vi "Habid_2-D_Histogram_Beta.vi"() -> ()   [LabVIEW 2009]
uses:
  <vilib>/Utility/file.llb/Write To Spreadsheet File (DBL).vi
  <vilib>/Analysis/3filter.llb/Butterworth Filter (DBL).vi
  <vilib>/Analysis/NI_AALBase.lvlib
  <vilib>/Analysis/NI_AALPro.lvlib
panel:
  in  "Save 2-D":bool
  in  "Result File Dir 2":path
  in  "Result File Name 2":string="1D_Histogram.txt"
  in  "Piezo Factor":dbl=0.88881
  out "SD":dbl[](array[numeric])
  in  "High Voltage Gain":dbl=5.0
  out "y-axis":dbl[](array[numeric])
  out "x-axis":dbl[](array[numeric])
  in  "Ramp Rate":dbl=5.0
  out "fit for M.A.":cluster{"Value":dbl, dbl, dbl[]}(graph)
  in  "Average Max?":bool
  out "Individual 2D Histogram":dbl[][](graph)
  out "Total 2D Histogram":dbl[][](graph)
  out "threshold":cluster{dbl, dbl, ext[]}(graph)
  out "Gain Multiplier I(t)":cluster{dbl, dbl, "Filtered X":dbl[]}(graph)
  out "After I(t)":cluster{dbl, dbl, "Filtered X":dbl[]}(graph)
  out "Before I(t)":cluster{dbl, "SamplingTime":dbl, "Data":ext[]}(graph)
  in  "start path":path=path "J:/data"
  out "NormAC":dbl[](array[numeric])
  in  "Save Curve?":bool
  out "CurrentFileName":string
  in  "Result File Name":string="1D_Histogram.txt"
  in  "Result File Dir":path
  in  "Save 1-D":bool
  out "SelectedCurves":i32
  out "CurvesInHistogram":bool[](array[boolean])
  in  "1-D Histogram?":bool
  in  "Continuous?":bool
  in  "Add Histogram?":bool
  in  "Beta bins":i32=100
  in  "Beta max":dbl=20.0
  in  "Beta min":dbl
  in  "Distance bins":i32=500
  in  "Distance max":dbl=4.0
  in  "Distance min":dbl
  in  "+/-":bool=TRUE
  out "DcData":dbl[](array[numeric])
  out "Beta":dbl[](array[numeric])
  out "DcDataLog":dbl[](array[numeric])
  out "TotalCurves":i32
  out "CurrentCurve":i32
  in  "Next Curve":bool
  in  "Previous Curve":bool
  out "AC I(t)":T1(graph)
  in  "Piezo Sensitivity (nm/V)":dbl=3.89
  in  "Z-mod Amp (V)":dbl=0.0257
  in  "Gac/Gdc":dbl=1.16618
  in  "low cutoff freq: fl":u32=600
  in  "high cutoff freq: fh":u32=1400
  out "DC I(t)":T2(graph)
  in  "DC cutoff freq":i32=1200
  out "Original I(t)":cluster{dbl, "SamplingTime":dbl, "Data":ext[]}(graph)
  out "DataBuffer":dbl[](array[numeric])
  out "Sampling Freq":dbl
  out "Sampling Time":dbl
  out "TimeLine":dbl[](array[numeric])
  in  "stop":bool
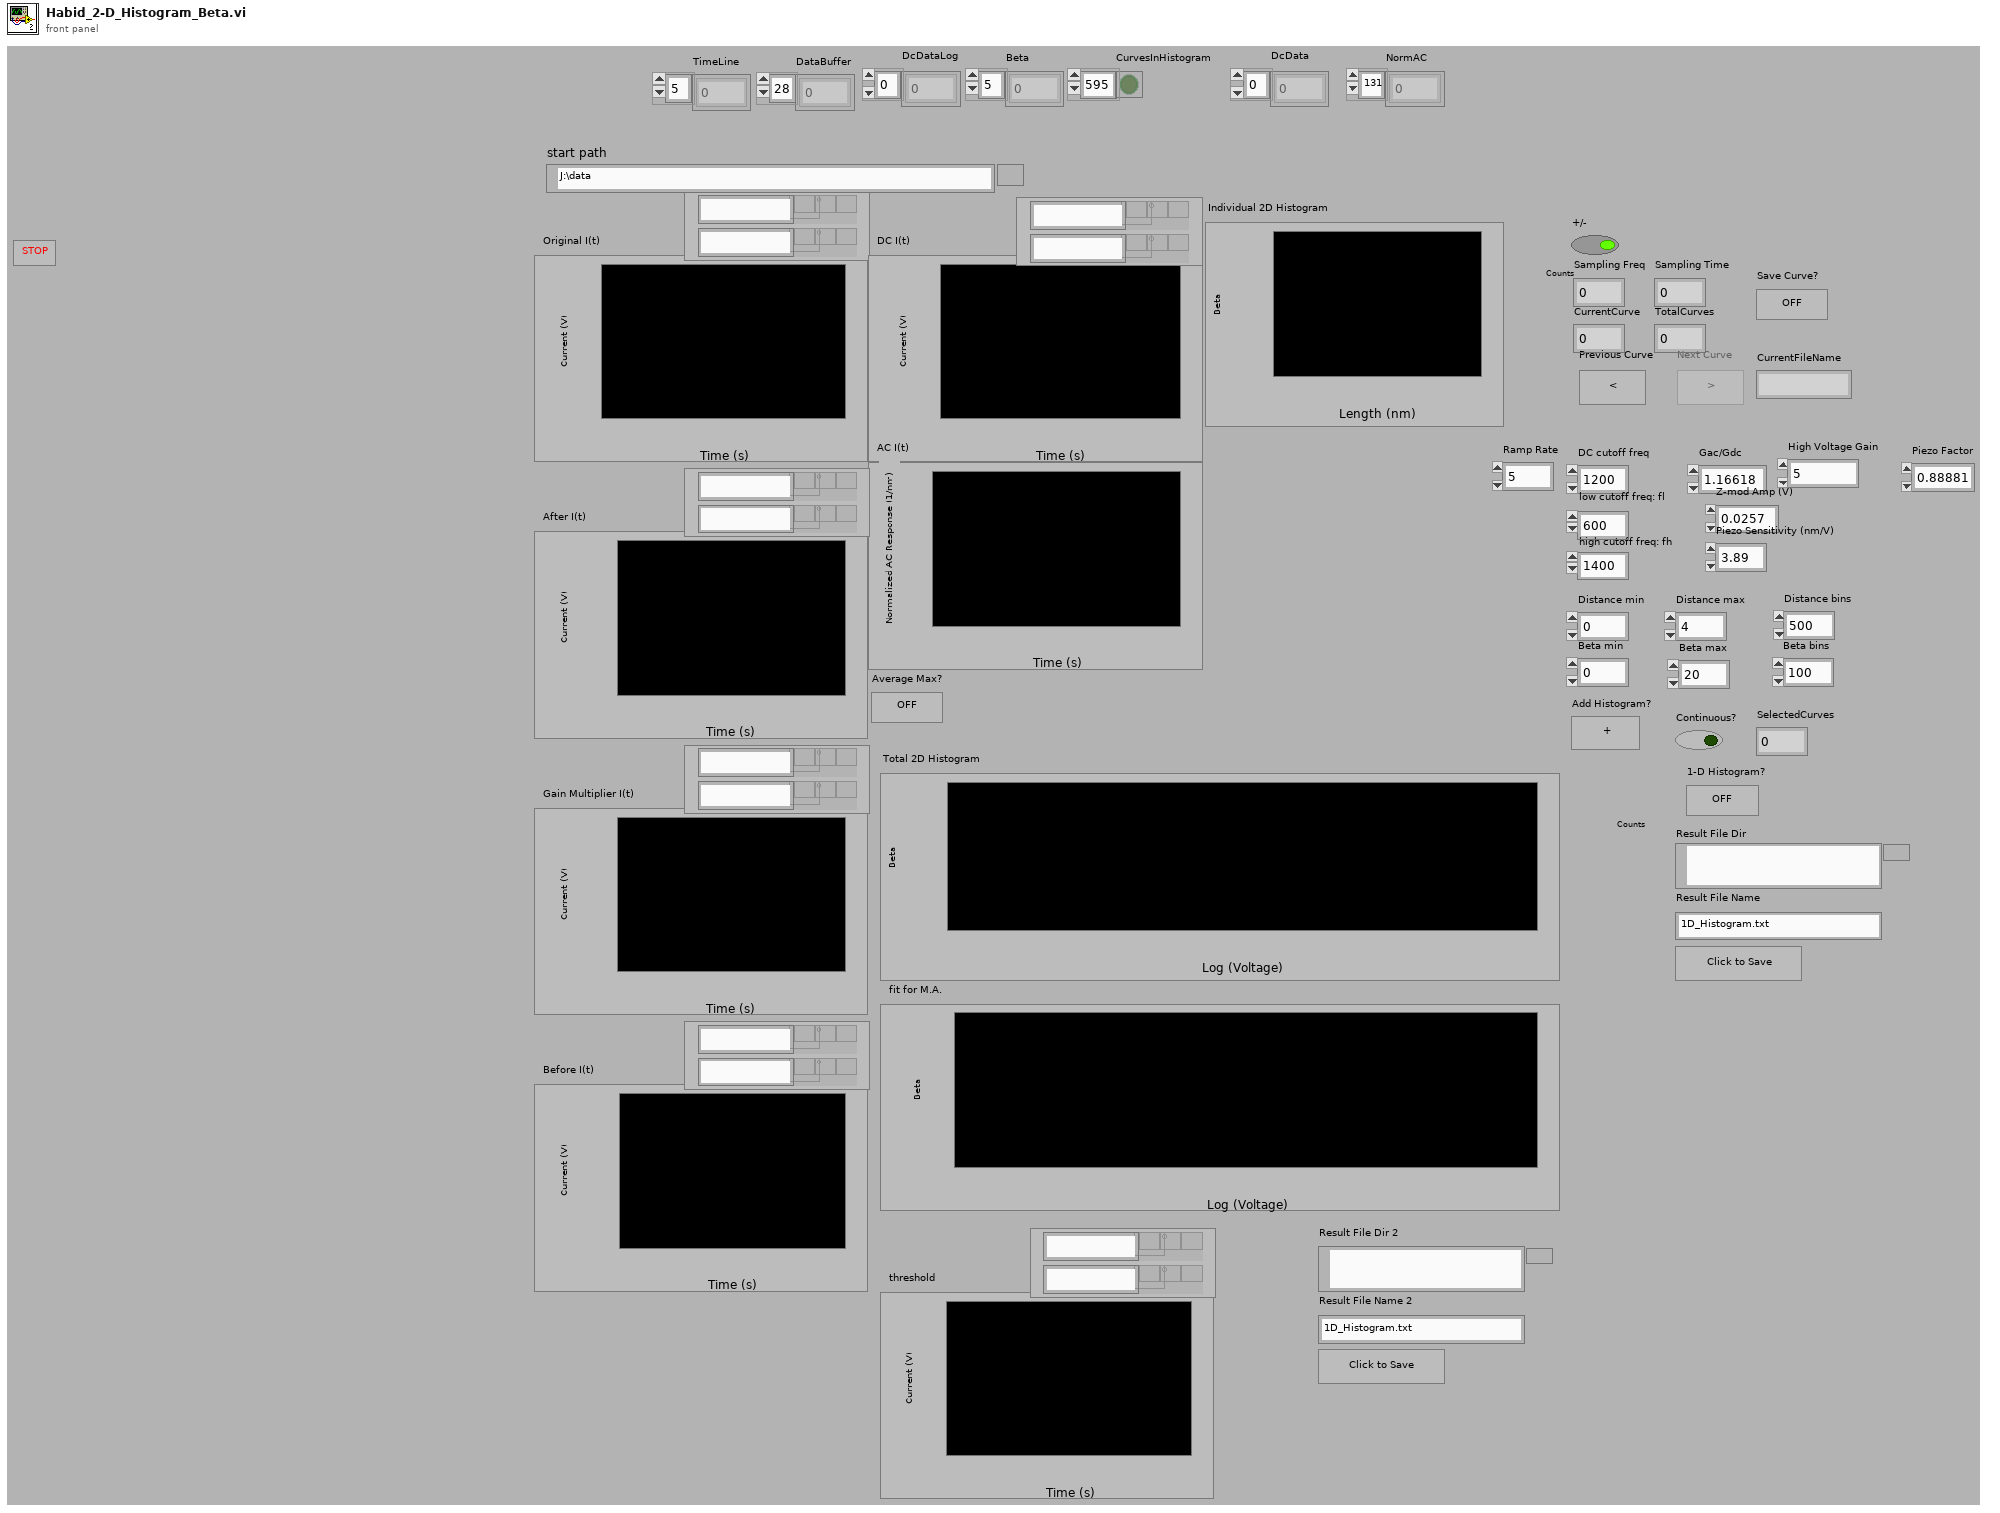
[diagram p1: front panel]
types:
  T1 = cluster{"Start Time":dbl, "Sampling Time":dbl, dbl[][]}
  T2 = cluster{dbl, "SamplingTime":dbl, "Filtered X":dbl[]}
  T3 = enum32{"Lowpass", "Highpass", "Bandpass", "Bandstop"}
  T4 = cluster{"Value":dbl, "XScale.Multiplier":dbl, dbl[]}
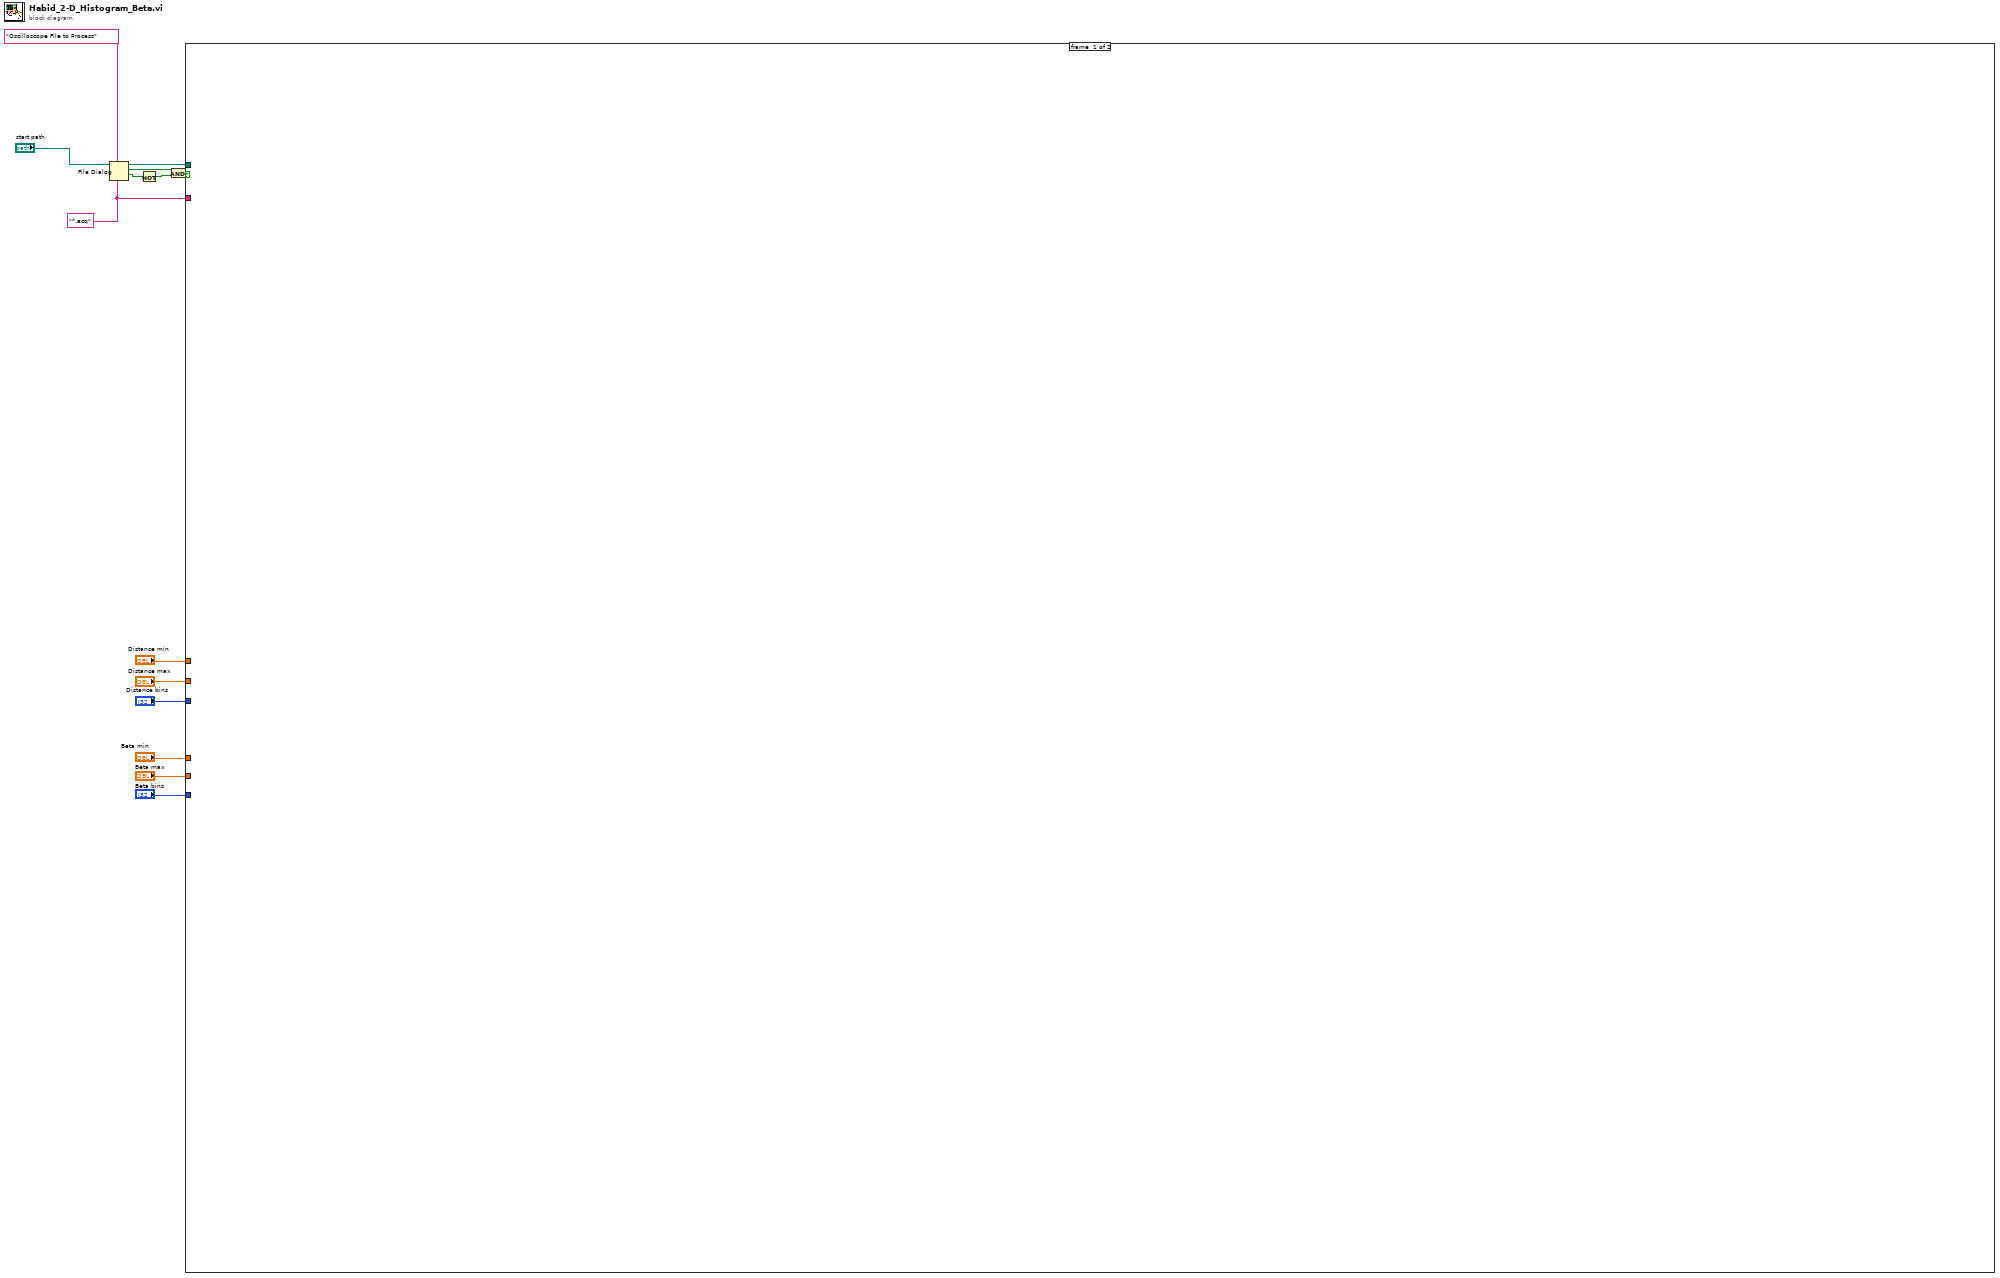
[diagram p0: block diagram]
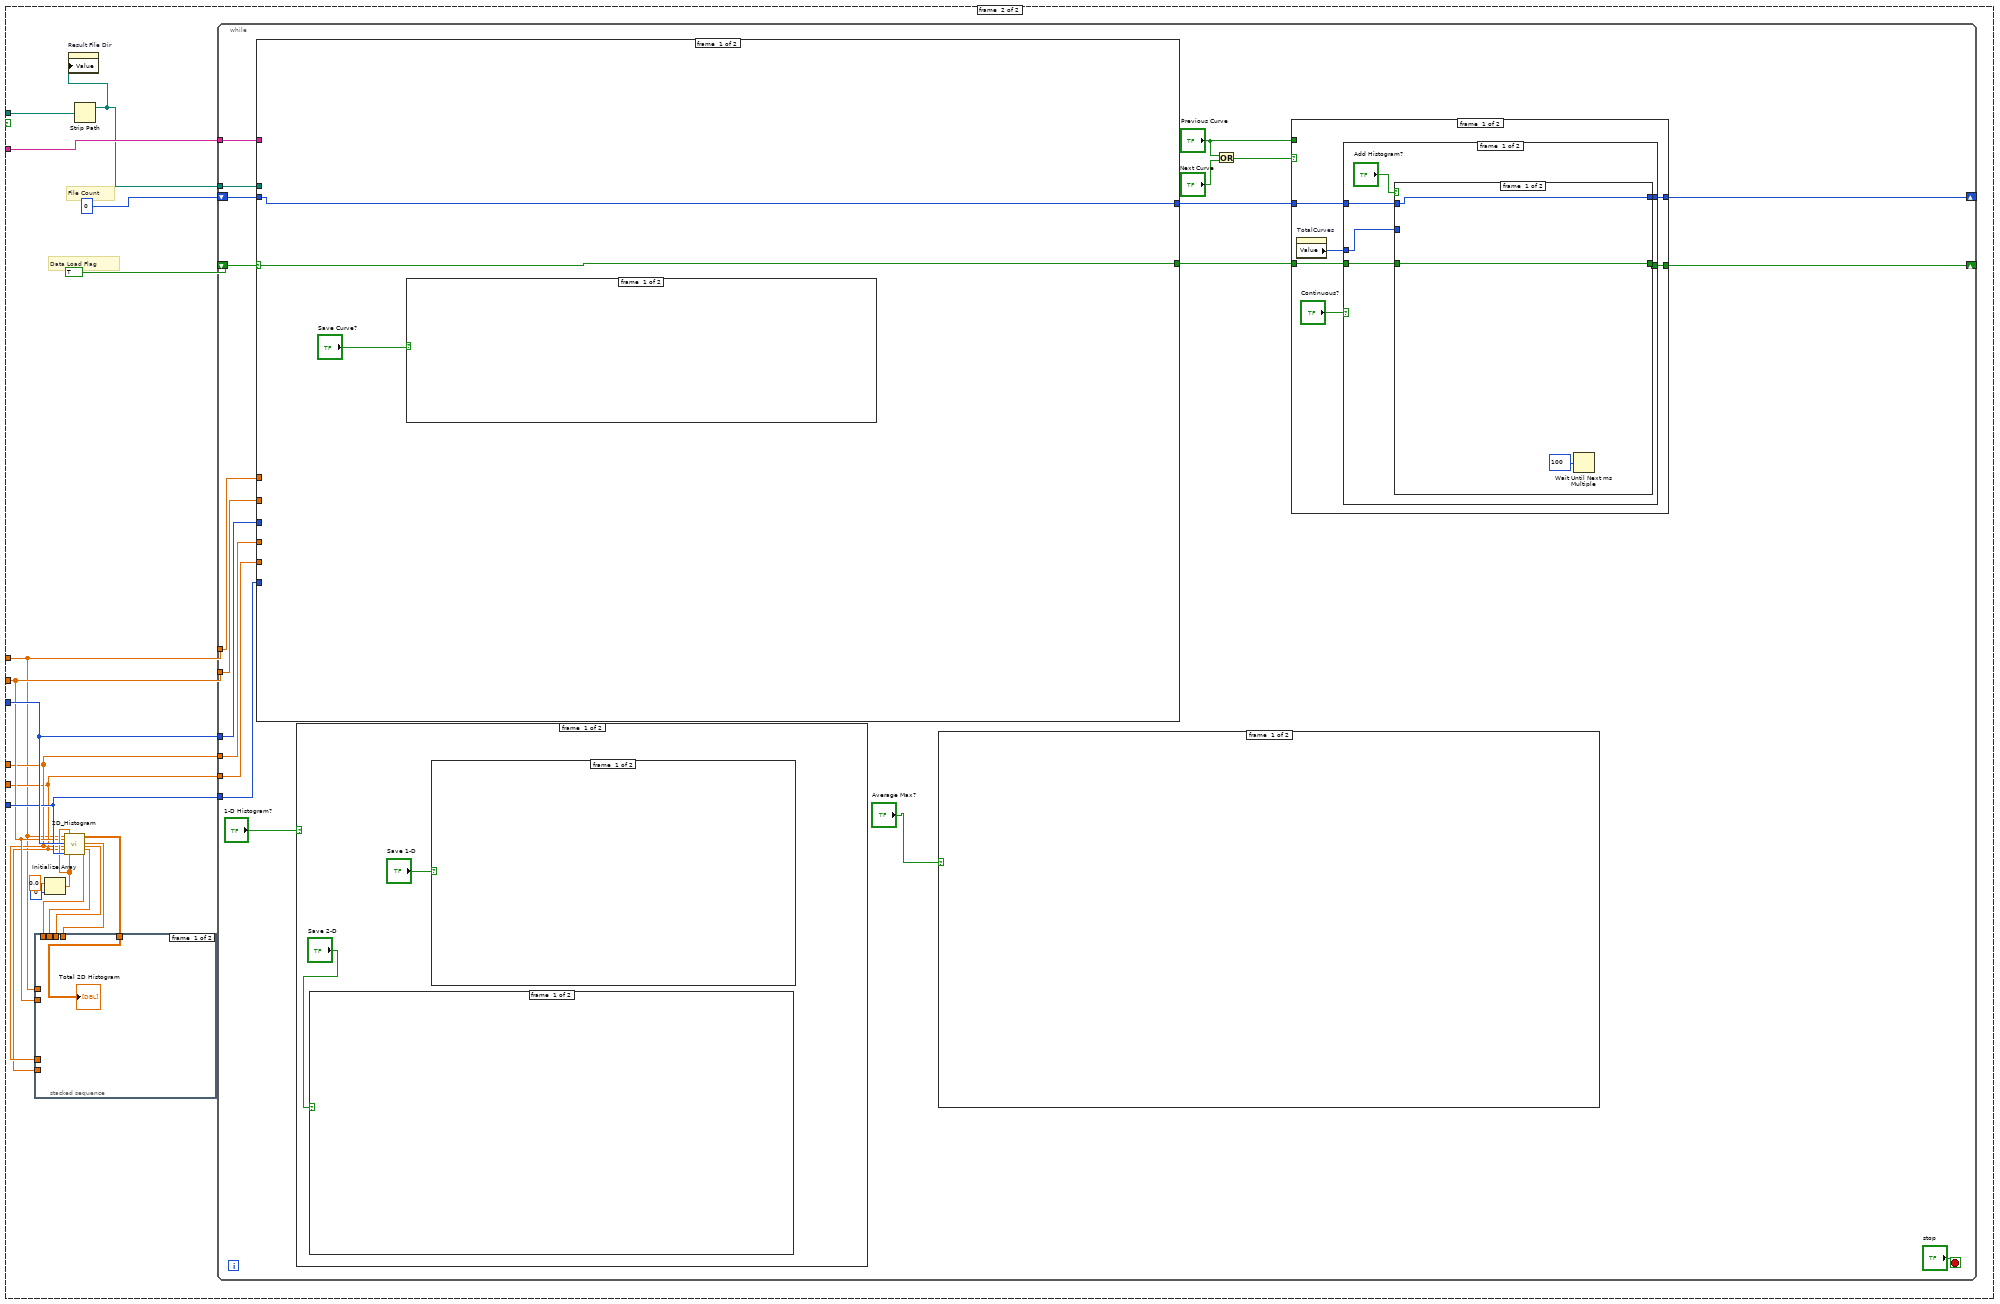
[diagram p2: hidden frame]
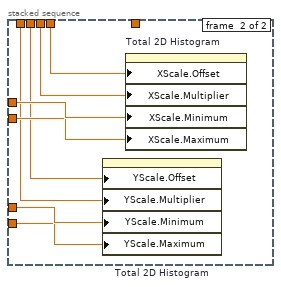
[diagram p3: hidden frame]
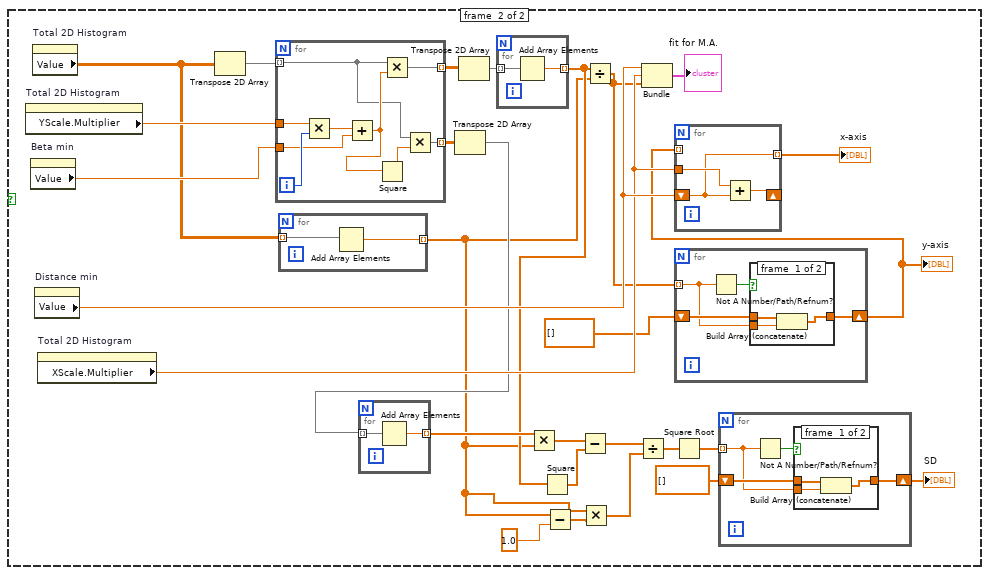
[diagram p4: hidden frame]
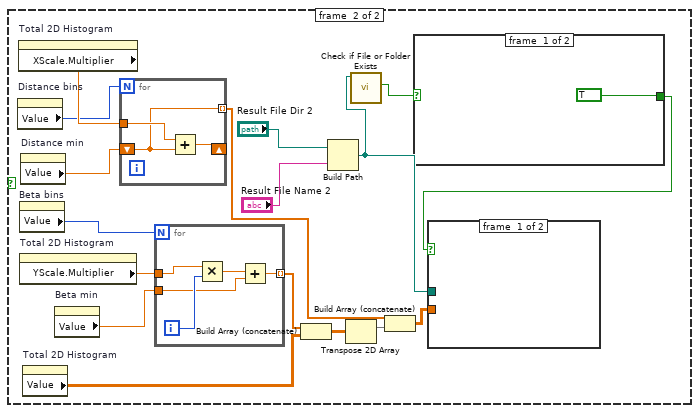
[diagram p7: hidden frame]
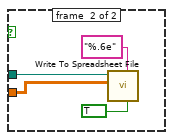
[diagram p8: hidden frame]
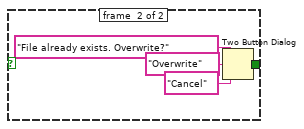
[diagram p9: hidden frame]
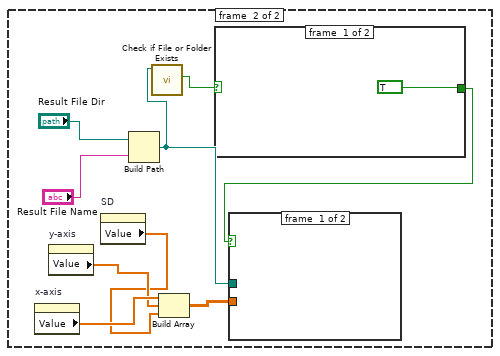
[diagram p10: hidden frame]
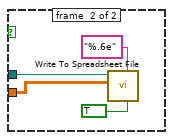
[diagram p11: hidden frame]
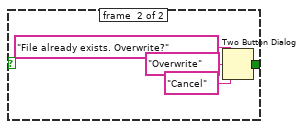
[diagram p12: hidden frame]
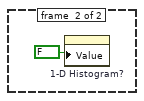
[diagram p13: hidden frame]
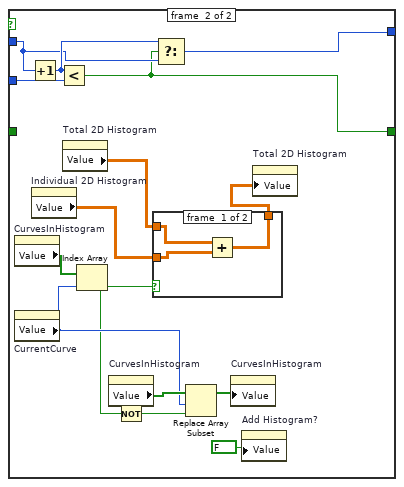
[diagram p14: hidden frame]
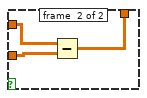
[diagram p15: hidden frame]
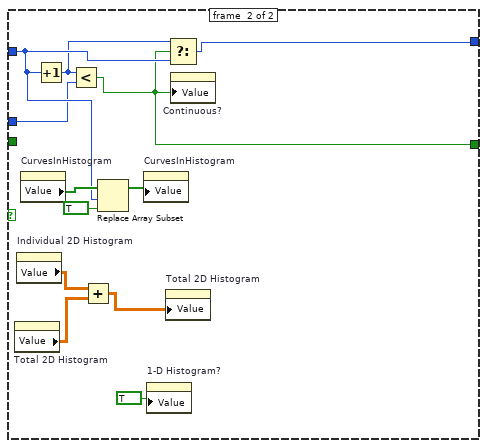
[diagram p16: hidden frame]
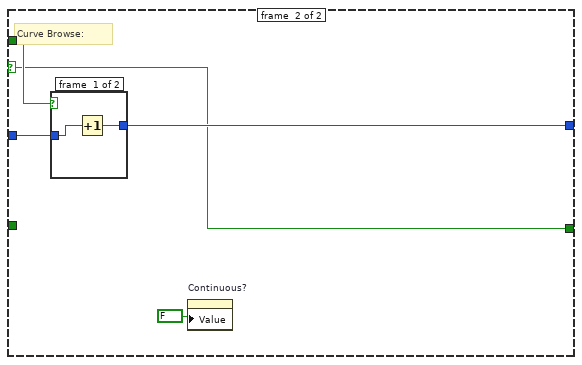
[diagram p17: hidden frame]
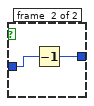
[diagram p18: hidden frame]
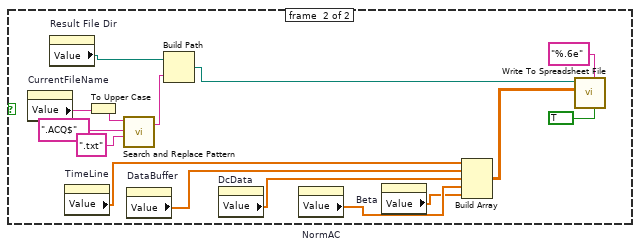
[diagram p19: hidden frame]
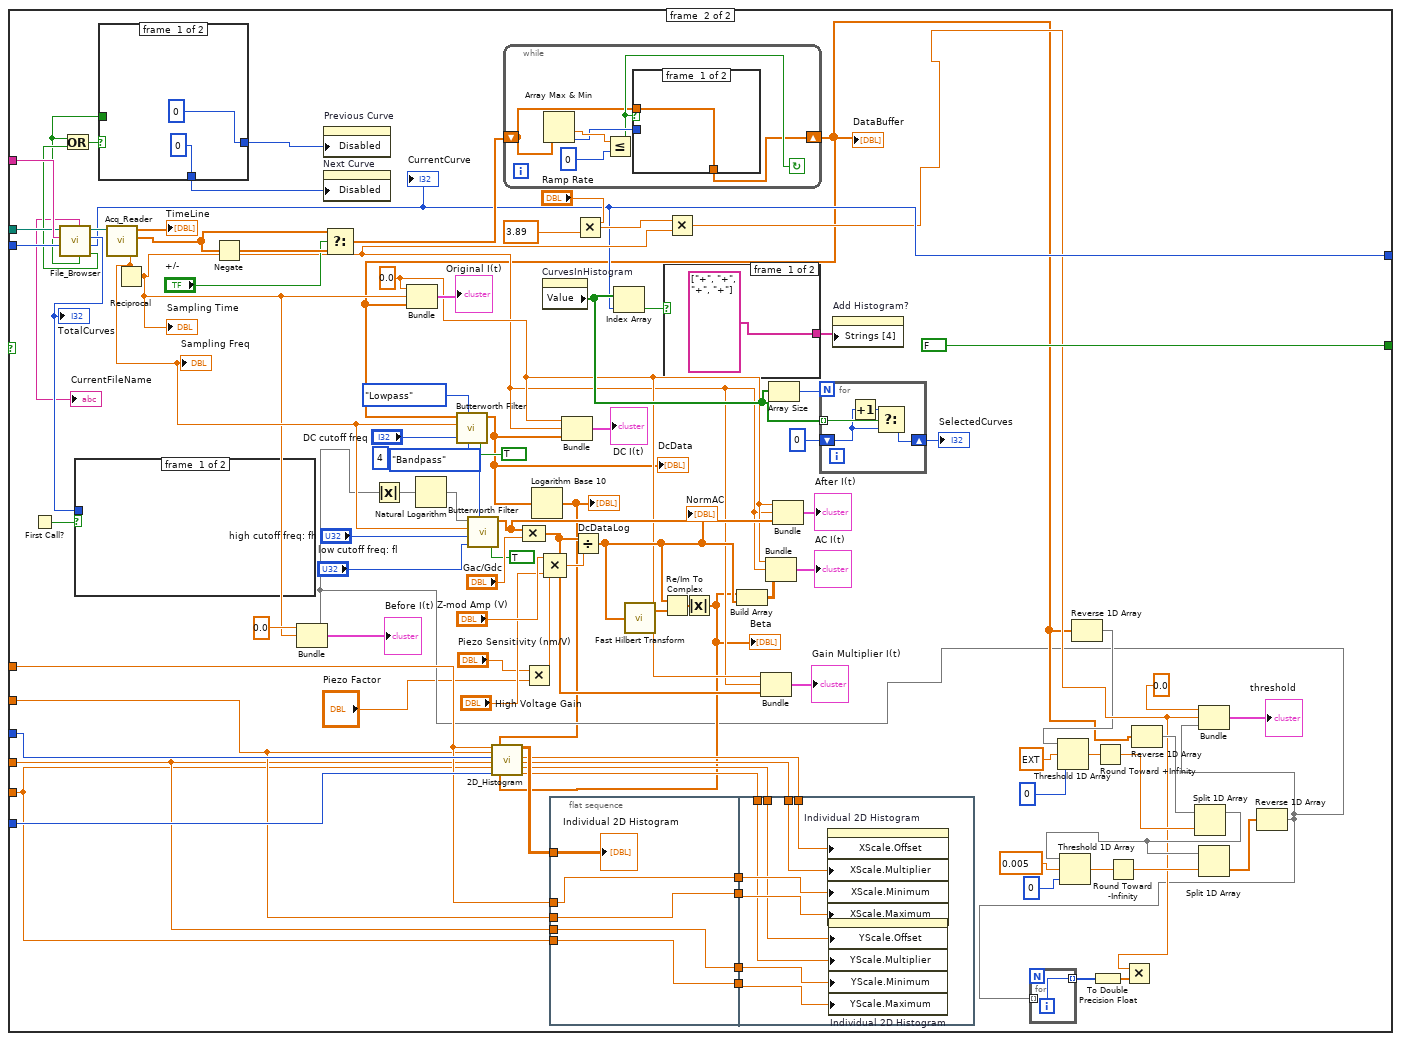
[diagram p20: hidden frame]
diagram:
  w7 = "*.acq" ("pattern (all files)")
  n1 = File Dialog(6:w7, 7:"Oscilloscope File to Process", 11:"start path") -> (1:w11:bool, 2:w13:bool, 3:w8:path)  [unwired: 4 in, 1 out]
  n2 = Not(x=w11) -> (.not. x?=w12:bool)
  n3 = And(x=w13, y=w12) -> (x .and. y?=w9:bool)
  n4 = case shown="True" w9 {
    tunnel: w8 -> [_ w33]
    tunnel: w7 -> [_ w31]
    tunnel: "Distance min" -> [_ w15]
    tunnel: "Distance max" -> [_ w18]
    tunnel: "Distance bins" -> [_ w29]
    tunnel: "Beta min" -> [_ w17]
    tunnel: "Beta max" -> [_ w16]
    tunnel: "Beta bins" -> [_ w28]
    frame #0 {
    }
    frame #1 {
      # "File Count"
      # "Data Load Flag"
      n5 = Initialize Array(0.0 ("element"), 0 ("dimension size")) -> (w20:dbl[])
      n6 = call "2D_Histogram.vi"("X min"=w15, "X max"=w18, "X bins"=w29, "Y min"=w17, "Y max"=w16, "Y bins"=w28, "X"=w20, "Y"=w20) -> ("X-Y 2-D Histogram"=w27:dbl[][], "Xoffset"=w26:dbl, "Xmultiplier"=w25:dbl, "Yoffset"=w24:dbl, "Ymultiplier"=w23:dbl)  [unwired: 7 in]
      n7 = stacked-sequence {
        tunnel: w27 -> [w34 _]
        tunnel: w25 -> [_ w41]
        tunnel: w23 -> [_ w37]
        tunnel: w26 -> [_ w42]
        tunnel: w24 -> [_ w38]
        tunnel: w15 -> [_ w40]
        tunnel: w18 -> [_ w39]
        tunnel: w17 -> [_ w36]
        tunnel: w16 -> [_ w35]
        frame #0 {
          "Total 2D Histogram" <- w34
        }
        frame #1 {
          n8 = property on="Total 2D Histogram" class="IntGraph (strict)"("YScale.Offset"=w38, "YScale.Multiplier"=w37, "YScale.Minimum"=w36, "YScale.Maximum"=w35) -> ()  [unwired: 2 in, 2 out]
          n9 = property on="Total 2D Histogram" class="IntGraph (strict)"("XScale.Offset"=w42, "XScale.Multiplier"=w41, "XScale.Minimum"=w40, "XScale.Maximum"=w39) -> ()  [unwired: 2 in, 2 out]
        }
      }
      n10 = Strip Path(path=w33) -> (stripped path=w19:path)  [unwired: 1 out]
      n11 = property on="Result File Dir" class="Path"("Value"=w19) -> ()  [unwired: 2 in, 2 out]
      n12 = while {
        shift-right: [w45] -> _
        shift-left: TRUE ("DataReload") -> [w61]
        tunnel: w31 -> [w60]
        tunnel: w19 -> [w59]
        shift-right: [w46] -> _
        shift-left: 0 -> [w58]
        tunnel: w15 -> [w55]
        tunnel: w18 -> [w54]
        tunnel: w29 -> [w53]
        tunnel: w17 -> [w52]
        tunnel: w16 -> [w51]
        tunnel: w28 -> [w50]
        stop <- "stop" stop-if-true
        n13 = case shown="True" w61 {
          selector: w61 -> [w239 _]
          tunnel: w60 -> [_ w352]
          tunnel: w59 -> [_ w351]
          tunnel: w58 -> [w238 w350]
          tunnel: [w239 FALSE] -> w57
          tunnel: [w238 w284] -> w56
          tunnel: w55 -> [_ w306]
          tunnel: w54 -> [_ w305]
          tunnel: w53 -> [_ w316]
          tunnel: w52 -> [_ w304]
          tunnel: w51 -> [_ w303]
          tunnel: w50 -> [_ w315]
          frame #0 {
            n14 = case shown="True" "Save Curve?" {
              frame #0 {
              }
              frame #1 {
                n15 = property on="CurrentFileName" class="Str"() -> ("Value"=w250:string)  [unwired: 2 in, 2 out]
                n16 = property on="Result File Dir" class="Path"() -> ("Value"=w254:path)  [unwired: 2 in, 2 out]
                n17 = property on="TimeLine" class="Arr (strict)"() -> ("Value"=w244:dbl[])  [unwired: 2 in, 2 out]
                n18 = To Upper Case(1:w250) -> (0:w251:string)
                n19 = call <vilib>:"Search and Replace Pattern.vi"("string"=w251, "regular expression (\"\")"=".ACQ$" ("regular expression (\"\")"), "replace string (\"\")"=".txt" ("replace string (\"\")")) -> ("result string"=w249:string)  [unwired: 2 in, 1 out]
                n20 = property on="DataBuffer" class="Arr (strict)"() -> ("Value"=w243:dbl[])  [unwired: 2 in, 2 out]
                n21 = Build Path(base path=w254, name or relative path=w249) -> (appended path=w246:path)
                n22 = property on="DcData" class="Arr (strict)"() -> ("Value"=w242:dbl[])  [unwired: 2 in, 2 out]
                n23 = property on="NormAC" class="Arr (strict)"() -> ("Value"=w241:dbl[])  [unwired: 2 in, 2 out]
                n24 = property on="Beta" class="Arr (strict)"() -> ("Value"=w240:dbl[])  [unwired: 2 in, 2 out]
                n25 = Build Array(w244, w243, w242, w241, w240) -> (w245:dbl[][])
                n26 = call-poly <vilib>:"Write To Spreadsheet File.vi"("transpose? (no:F)"=TRUE, "format (%.3f)"="%.6e", "2D data"=w245, "file path (dialog if empty)"=w246) -> ()  [unwired: 4 in, 1 out]
              }
            }
          }
          frame #1 {
            w290 = 0.0
            n27 = First Call?() -> (First Call?: T/F=w314:bool)
            n28 = call "File_Browser.vi"("FileIndexIn"=w350, "FileExt"=w352, "FolderPath"=w351) -> ("Last?"=w328:bool, "FileIndexOut"=w284:i32, "FileTotal"=w313:i32, "FullFilePath"=w349:path, "First?"=w327:bool, "FileName"=→"CurrentFileName":string)  [unwired: 3 in]
            "CurrentCurve" <- w284
            "TotalCurves" <- w313
            n29 = Or(x=w327, y=w328) -> (x .or. y?=w331:bool)
            n30 = case shown="True" w314 {
              tunnel: w313 -> [_ w361]
              frame #0 {
              }
              frame #1 {
                n31 = Initialize Array(FALSE ("DataReload"), w361) -> (→"CurvesInHistogram":bool[])
              }
            }
            n32 = case shown="True" w331 {
              tunnel: w327 -> [_ w391]
              tunnel: [0 w390] -> w329
              tunnel: [0 w389] -> w330
              frame #0 {
              }
              frame #1 {
                # "Button Control:"
                n33 = case shown="True" w391 {
                  tunnel: [0 2] -> w390
                  tunnel: [2 0] -> w389
                  frame #0 {
                  }
                  frame #1 {
                  }
                }
              }
            }
            n34 = call "Acq_Reader.vi"("AcqFileToRead"=w349) -> ("SamplingFreq"=w326:dbl, "Data"=w324:ext[], "TimeLine"=→"TimeLine":dbl[])  [unwired: 8 in]
            "Sampling Freq" <- w326
            n35 = Reciprocal(x=w326) -> (1/x=w285:dbl)
            "Sampling Time" <- w285
            n36 = Negate(x=w324) -> (-x=w323:ext[])
            n37 = property on="Previous Curve" class="Bool"("Disabled"=w329) -> ()  [unwired: 2 in, 2 out]
            n38 = property on="Next Curve" class="Bool"("Disabled"=w330) -> ()  [unwired: 2 in, 2 out]
            n39 = Select(t=w324, s="+/-", f=w323) -> (s? t:f=w325:ext[])
            n40 = while {
              shift-right: [w376] -> w264
              shift-left: w325 -> [w377]
              stop <- w378 continue-if-true
              n41 = Array Max & Min(array=w377) -> (min value=w380:ext, min index (indices)=w379:i32)  [unwired: 2 out]
              n42 = Less Or Equal?(x=w380, y=0) -> (x <= y?=w378:bool)
              n43 = case shown="True" w378 {
                tunnel: w379 -> [_ w386]
                tunnel: w377 -> [w382 w385]
                tunnel: [w382 w384] -> w376
                frame #0 {
                }
                frame #1 {
                  n44 = Replace Array Subset(array=w385, new element=ext 0.00000100000000000000000004 ("new element/subarray"), index=w386) -> (w384:ext[])
                }
              }
            }
            "DataBuffer" <- w264
            n45 = Bundle(w290, w285, "Data"=w264) -> (→"Original I(t)":cluster{dbl, dbl, "Data":ext[]})  [unwired: 1 in]
            n46 = call-poly <vilib>:"Butterworth Filter.vi"("init/cont (init:F)"=TRUE, "order"=4, "filter type"=T3."Lowpass", "low cutoff freq: fl"="DC cutoff freq", "sampling freq: fs"=w326, "X"=w264) -> ("Filtered X"=w265:dbl[])  [unwired: 2 in, 1 out]
            "DcData" <- w265
            n47 = Multiply(x="Piezo Sensitivity (nm/V)", y="Piezo Factor") -> (x*y=w257:dbl)
            n48 = Logarithm Base 10(1:w265) -> (0:w255:dbl[])
            "DcDataLog" <- w255
            n49 = property on="CurvesInHistogram" class="Arr (strict)"() -> ("Value"=w308:bool[])  [unwired: 2 in, 2 out]
            n50 = Compound Arithmetic op=MULTIPLY("Z-mod Amp (V)", w257, "High Voltage Gain") -> (w338:dbl)
            n51 = flat-sequence {
              tunnel: w321 -> [w363]
              tunnel: w306 -> [w367]
              tunnel: w305 -> [w366]
              tunnel: w304 -> [w365]
              tunnel: w303 -> [w364]
              tunnel: [w367] -> w302
              tunnel: [w366] -> w301
              tunnel: [w365] -> w300
              tunnel: [w364] -> w299
              tunnel: w320 -> [w374]
              tunnel: w319 -> [w370]
              tunnel: w318 -> [w375]
              tunnel: w317 -> [w371]
              tunnel: w302 -> [w373]
              tunnel: w301 -> [w372]
              tunnel: w300 -> [w369]
              tunnel: w299 -> [w368]
              frame #0 {
                "Individual 2D Histogram" <- w363
              }
              frame #1 {
                n52 = property on="Individual 2D Histogram" class="IntGraph (strict)"("XScale.Offset"=w375, "XScale.Multiplier"=w374, "XScale.Minimum"=w373, "XScale.Maximum"=w372) -> ()  [unwired: 2 in, 2 out]
                n53 = property on="Individual 2D Histogram" class="IntGraph (strict)"("YScale.Offset"=w371, "YScale.Multiplier"=w370, "YScale.Minimum"=w369, "YScale.Maximum"=w368) -> ()  [unwired: 2 in, 2 out]
              }
            }
            n54 = Bundle(w290, w285, "Filtered X"=w265) -> (→"DC I(t)":cluster{dbl, dbl, "Filtered X":dbl[]})  [unwired: 1 in]
            n55 = Multiply(x="Ramp Rate", y=3.89) -> (x*y=w286:dbl)
            n56 = Index Array(array=w308, index=w284) -> (element=w312:bool)
            n57 = case shown="False" w312 {
              tunnel: [string[] ["+", "+", "+", "+"] ("Strings [4]") string[] ["-", "-", "-", "-"] ("Strings [4]")] -> w311
              frame #0 {
              }
              frame #1 {
              }
            }
            n58 = Multiply(x=w286, y=w285) -> (x*y=w268:dbl)
            n59 = Array Size(array=w308) -> (size(s)=w310:i32)
            n60 = for {
              N: w310 -> [_]
              shift-right: [w354] -> w307
              shift-left: 0 -> [w356]
              tunnel: w308 -> [w357] mode=indexing
              n61 = Increment(x=w356) -> (x+1=w355:i32)
              n62 = Select(t=w355, s=w357, f=w356) -> (s? t:f=w354:i32)
            }
            "SelectedCurves" <- w307
            n63 = property on="Add Histogram?" class="Bool (strict)"("Strings [4]"=w311) -> ()  [unwired: 2 in, 2 out]
            n64 = Reverse 1D Array(array=w264) -> (reversed array=w267:ext[])
            n65 = Threshold 1D Array(1:0 ("start index (0)"), 2:ext 10.0 ("threshold y"), 3:w267) -> (0:w278:ext)
            n66 = Round Toward +Infinity(x=w278) -> (ceil(x): smallest int >= x=w279:ext)
            n67 = Reverse 1D Array(array=w264) -> (reversed array=w280:ext[])
            n68 = Split 1D Array(array=w280, index=w279) -> (first subarray=w276:ext[])  [unwired: 1 out]
            n69 = Threshold 1D Array(1:0 ("start index (0)"), 2:0.005 ("threshold y"), 3:w276) -> (0:w273:ext)
            n70 = Round Toward -Infinity(1:w273) -> (0:w272:ext)
            n71 = Split 1D Array(array=w276, index=w272) -> (second subarray=w275:ext[])  [unwired: 1 out]
            n72 = Reverse 1D Array(array=w275) -> (reversed array=w260:ext[])
            n73 = Bundle(0.0, w285, w260) -> (→"Before I(t)":cluster{dbl, dbl, ext[]})  [unwired: 1 in]
            n74 = Absolute Value(x=w260) -> (abs(x)=w262:ext[])
            n75 = Natural Logarithm(1:w262) -> (0:w261:ext[])
            n76 = call-poly <vilib>:"Butterworth Filter.vi"("init/cont (init:F)"=TRUE, "filter type"=T3."Bandpass", "low cutoff freq: fl"="low cutoff freq: fl", "high cutoff freq: fh"="high cutoff freq: fh", "sampling freq: fs"=w326, "X"=w261) -> ("Filtered X"=w292:dbl[])  [unwired: 2 in, 1 out]
            n77 = Compound Arithmetic op=MULTIPLY(w292, "Gac/Gdc") -> (w289:dbl[])
            n78 = Divide(x=w289, y=w338) -> (x/y=w333:dbl[])
            "NormAC" <- w333
            n79 = call <vilib>:"Fast Hilbert Transform.vi"("X"=w333) -> ("Hilbert{X}"=w337:dbl[])  [unwired: 1 out]
            n80 = Re/Im To Complex(1:w337, 2:w333) -> (0:w336:cdb[])
            n81 = Absolute Value(x=w336) -> (abs(x)=w263:dbl[])
            "Beta" <- w263
            n82 = call "2D_Histogram.vi"("X min"=w306, "X max"=w305, "X bins"=w316, "Y min"=w304, "Y max"=w303, "Y bins"=w315, "X"=w255, "Y"=w263) -> ("X-Y 2-D Histogram"=w321:dbl[][], "Xoffset"=w318:dbl, "Xmultiplier"=w320:dbl, "Yoffset"=w317:dbl, "Ymultiplier"=w319:dbl)  [unwired: 7 in]
            n83 = Build Array(w263, w333) -> (w335:dbl[][])
            n84 = Bundle(w290, w285, w289) -> (→"Gain Multiplier I(t)":cluster{dbl, dbl, dbl[]})  [unwired: 1 in]
            n85 = Bundle(w290, w285, w335) -> (→"AC I(t)":cluster{dbl, dbl, dbl[][]})  [unwired: 1 in]
            n86 = Bundle(w290, w285, "Filtered X"=w292) -> (→"After I(t)":cluster{dbl, dbl, "Filtered X":dbl[]})  [unwired: 1 in]
            n87 = for {
              tunnel: [w353] -> w271 mode=indexing
              tunnel: w260 -> [_] mode=indexing
              i -> [w353]
            }
            n88 = To Double Precision Float(number=w271) -> (double precision float=w270:dbl[])
            n89 = Multiply(x=w268, y=w270) -> ()  [unwired: 1 out]
            n90 = Bundle(0.0, w268, w260) -> (→"threshold":cluster{dbl, dbl, ext[]})  [unwired: 1 in]
          }
        }
        n91 = case shown="False" "1-D Histogram?" {
          frame #0 {
            n92 = case shown="True" "Save 2-D" {
              frame #0 {
              }
              frame #1 {
                n93 = property on="Distance bins" class="DigNum (strict)"() -> ("Value"=w134:i32)  [unwired: 2 in, 2 out]
                n94 = property on="Total 2D Histogram" class="IntGraph (strict)"() -> ("XScale.Multiplier"=w135:dbl)  [unwired: 2 in, 2 out]
                n95 = property on="Beta bins" class="DigNum (strict)"() -> ("Value"=w138:i32)  [unwired: 2 in, 2 out]
                n96 = property on="Total 2D Histogram" class="IntGraph (strict)"() -> ("YScale.Multiplier"=w137:dbl)  [unwired: 2 in, 2 out]
                n97 = property on="Distance min" class="DigNum (strict)"() -> ("Value"=w133:dbl)  [unwired: 2 in, 2 out]
                n98 = property on="Total 2D Histogram" class="IntGraph (strict)"() -> ("Value"=w132:dbl[][])  [unwired: 2 in, 2 out]
                n99 = property on="Beta min" class="DigNum (strict)"() -> ("Value"=w136:dbl)  [unwired: 2 in, 2 out]
                n100 = for {
                  N: w134 -> [_]
                  tunnel: w135 -> [w146]
                  shift-right: [w145] -> _
                  shift-left: w133 -> [w144]
                  tunnel: [w144] -> w128 mode=indexing
                  n101 = Add(x=w146, y=w144) -> (x+y=w145:dbl)
                }
                n102 = for {
                  N: w138 -> [_]
                  tunnel: w137 -> [w149]
                  tunnel: w136 -> [w148]
                  tunnel: [w147] -> w131 mode=indexing
                  i -> [w150]
                  n103 = Multiply(x=w149, y=w150) -> (x*y=w151:dbl)
                  n104 = Add(x=w151, y=w148) -> (x+y=w147:dbl)
                }
                n105 = Build Array (concatenate)(w131, w132) -> (w130:dbl[][])
                n106 = Build Path(base path="Result File Dir 2", name or relative path="Result File Name 2") -> (appended path=w139:path)
                n107 = Transpose 2D Array(2D array=w130) -> (transposed array=w129:dbl[][])
                n108 = call <vilib>:"Check if File or Folder Exists.vi"("path"=w139) -> ("file or folder exists?"=w141:bool)  [unwired: 8 in, 2 out]
                n109 = Build Array (concatenate)(w128, w129) -> (w127:dbl[][])
                n110 = case shown="True" w141 {
                  tunnel: [TRUE ("T button?") w157] -> w140
                  frame #0 {
                  }
                  frame #1 {
                    n111 = Two Button Dialog(message="File already exists. Overwrite?", 1:"Cancel" ("F button name (\"Cancel\")"), 2:"Overwrite" ("T button name (\"OK\")")) -> (T button?=w157:bool)
                  }
                }
                n112 = case shown="True" w140 {
                  tunnel: w139 -> [_ w154]
                  tunnel: w127 -> [_ w152]
                  frame #0 {
                  }
                  frame #1 {
                    n113 = call-poly <vilib>:"Write To Spreadsheet File.vi"("transpose? (no:F)"=TRUE, "format (%.3f)"="%.6e", "2D data"=w152, "file path (dialog if empty)"=w154) -> ()  [unwired: 4 in, 1 out]
                  }
                }
              }
            }
            n114 = case shown="True" "Save 1-D" {
              frame #0 {
              }
              frame #1 {
                n115 = property on="x-axis" class="Arr (strict)"() -> ("Value"=w164:dbl[])  [unwired: 2 in, 2 out]
                n116 = property on="y-axis" class="Arr (strict)"() -> ("Value"=w162:dbl[])  [unwired: 2 in, 2 out]
                n117 = property on="SD" class="Arr (strict)"() -> ("Value"=w161:dbl[])  [unwired: 2 in, 2 out]
                n118 = Build Path(base path="Result File Dir", name or relative path="Result File Name") -> (appended path=w165:path)
                n119 = call <vilib>:"Check if File or Folder Exists.vi"("path"=w165) -> ("file or folder exists?"=w167:bool)  [unwired: 8 in, 2 out]
                n120 = Build Array(w164, w162, w161) -> (w163:dbl[][])
                n121 = case shown="True" w167 {
                  tunnel: [TRUE ("T button?") w175] -> w166
                  frame #0 {
                  }
                  frame #1 {
                    n122 = Two Button Dialog(message="File already exists. Overwrite?", 1:"Cancel" ("F button name (\"Cancel\")"), 2:"Overwrite" ("T button name (\"OK\")")) -> (T button?=w175:bool)
                  }
                }
                n123 = case shown="True" w166 {
                  tunnel: w165 -> [_ w172]
                  tunnel: w163 -> [_ w170]
                  frame #0 {
                  }
                  frame #1 {
                    n124 = call-poly <vilib>:"Write To Spreadsheet File.vi"("transpose? (no:F)"=TRUE, "format (%.3f)"="%.6e", "2D data"=w170, "file path (dialog if empty)"=w172) -> ()  [unwired: 4 in, 1 out]
                  }
                }
              }
            }
          }
          frame #1 {
            n125 = property on="1-D Histogram?" class="Bool (strict)"("Value"=FALSE ("1-D Histogram?")) -> ()  [unwired: 2 in, 2 out]
          }
        }
        n126 = case shown="True" "Average Max?" {
          frame #0 {
          }
          frame #1 {
            n127 = property on="Total 2D Histogram" class="IntGraph (strict)"() -> ("YScale.Multiplier"=w89:dbl)  [unwired: 2 in, 2 out]
            n128 = property on="Beta min" class="DigNum (strict)"() -> ("Value"=w88:dbl)  [unwired: 2 in, 2 out]
            n129 = property on="Total 2D Histogram" class="IntGraph (strict)"() -> ("Value"=w87:dbl[][])  [unwired: 2 in, 2 out]
            n130 = property on="Distance min" class="DigNum (strict)"() -> ("Value"=w83:dbl)  [unwired: 2 in, 2 out]
            n131 = property on="Total 2D Histogram" class="IntGraph (strict)"() -> ("XScale.Multiplier"=w82:dbl)  [unwired: 2 in, 2 out]
            n132 = Transpose 2D Array(2D array=w87) -> (transposed array=w90:dbl[][])
            n133 = for {
              tunnel: w90 -> [w117] mode=indexing
              tunnel: w89 -> [w123]
              tunnel: w88 -> [w121]
              tunnel: [w120] -> w86 mode=indexing
              tunnel: [w116] -> w77 mode=indexing
              i -> [w124]
              n134 = Multiply(x=w123, y=w124) -> (x*y=w122:dbl)
              n135 = Add(x=w122, y=w121) -> (x+y=w119:dbl)
              n136 = Square(x=w119) -> (x^2=w118:dbl)
              n137 = Multiply(x=w117, y=w119) -> (x*y=w120:dbl[])
              n138 = Multiply(x=w117, y=w118) -> (x*y=w116:dbl[])
            }
            n139 = for {
              tunnel: w87 -> [w115] mode=indexing
              tunnel: [w114] -> w69 mode=indexing
              n140 = Add Array Elements(numeric array=w115) -> (sum=w114:dbl)
            }
            n141 = Transpose 2D Array(2D array=w77) -> (transposed array=w76:dbl[][])
            n142 = for {
              tunnel: w76 -> [w100] mode=indexing
              tunnel: [w99] -> w75 mode=indexing
              n143 = Add Array Elements(numeric array=w100) -> (sum=w99:dbl)
            }
            n144 = Transpose 2D Array(2D array=w86) -> (transposed array=w85:dbl[][])
            n145 = for {
              tunnel: w85 -> [w113] mode=indexing
              tunnel: [w112] -> w73 mode=indexing
              n146 = Add Array Elements(numeric array=w113) -> (sum=w112:dbl)
            }
            n147 = Multiply(x=w75, y=w69) -> (x*y=w74:dbl[])
            n148 = Square(x=w73) -> (x^2=w72:dbl[])
            n149 = Subtract(x=w69, y=1.0) -> (x-y=w70:dbl[])
            n150 = Subtract(x=w74, y=w72) -> (x-y=w68:dbl[])
            n151 = Multiply(x=w69, y=w70) -> (x*y=w67:dbl[])
            n152 = Divide(x=w73, y=w69) -> (x/y=w80:dbl[])
            n153 = Divide(x=w68, y=w67) -> (x/y=w66:dbl[])
            n154 = Bundle("Value"=w83, "XScale.Multiplier"=w82, w80) -> (→"fit for M.A.":T4)  [unwired: 1 in]
            n155 = Square Root(x=w66) -> (sqrt(x)=w65:dbl[])
            n156 = for {
              tunnel: w80 -> [w101] mode=indexing
              shift-right: [w102] -> w78
              shift-left: dbl[] [] ("Arrayin 2") -> [w103]
              n157 = Not A Number/Path/Refnum?(number/path/refnum=w101) -> (NaN/Path/Refnum?=w104:bool)
              n158 = case shown="True" w104 {
                tunnel: w103 -> [w107 w108]
                tunnel: [w106 w108] -> w102
                tunnel: w101 -> [w105 _]
                frame #0 {
                  n159 = Build Array (concatenate)(w107, w105) -> (w106:dbl[])
                }
                frame #1 {
                }
              }
            }
            "y-axis" <- w78
            n160 = for {
              tunnel: w82 -> [w111]
              shift-right: [w110] -> _
              shift-left: w83 -> [w109]
              tunnel: [w109] -> w81 mode=indexing
              tunnel: w78 -> [_] mode=indexing
              n161 = Add(x=w111, y=w109) -> (x+y=w110:dbl)
            }
            "x-axis" <- w81
            n162 = for {
              tunnel: w65 -> [w91] mode=indexing
              shift-right: [w92] -> w63
              shift-left: dbl[] [] -> [w93]
              n163 = Not A Number/Path/Refnum?(number/path/refnum=w91) -> (NaN/Path/Refnum?=w94:bool)
              n164 = case shown="True" w94 {
                tunnel: w93 -> [w97 w98]
                tunnel: [w96 w98] -> w92
                tunnel: w91 -> [w95 _]
                frame #0 {
                  n165 = Build Array (concatenate)(w97, w95) -> (w96:dbl[])
                }
                frame #1 {
                }
              }
            }
            "SD" <- w63
          }
        }
        n166 = Or(x="Previous Curve", y="Next Curve") -> (x .or. y?=w48:bool)
        n167 = case shown="False" w48 {
          selector: w48 -> [_ w229]
          tunnel: "Previous Curve" -> [_ w232]
          tunnel: w56 -> [w182 w231]
          tunnel: [w181 w230] -> w46
          tunnel: w57 -> [w185 _]
          tunnel: [w184 w229] -> w45
          frame #0 {
            n168 = property on="TotalCurves" class="DigNum (strict)"() -> ("Value"=w180:i32)  [unwired: 2 in, 2 out]
            n169 = case shown="False" "Continuous?" {
              tunnel: w185 -> [w188 _]
              tunnel: [w187 w219] -> w184
              tunnel: w182 -> [w190 w224]
              tunnel: [w189 w227] -> w181
              tunnel: w180 -> [w186 w221]
              frame #0 {
                n170 = case shown="True" "Add Histogram?" {
                  tunnel: w190 -> [w194 w200]
                  tunnel: [w194 w199] -> w189
                  tunnel: w188 -> [w193 _]
                  tunnel: [w193 w198] -> w187
                  tunnel: w186 -> [_ w202]
                  frame #0 {
                    n171 = Wait Until Next ms Multiple(millisecond multiple=u32 100) -> ()  [unwired: 1 out]
                  }
                  frame #1 {
                    n172 = property on="CurvesInHistogram" class="Arr (strict)"() -> ("Value"=w208:bool[])  [unwired: 2 in, 2 out]
                    n173 = property on="CurrentCurve" class="DigNum (strict)"() -> ("Value"=w205:i32)  [unwired: 2 in, 2 out]
                    n174 = Increment(x=w200) -> (x+1=w201:i32)
                    n175 = property on="Individual 2D Histogram" class="IntGraph (strict)"() -> ("Value"=w195:dbl[][])  [unwired: 2 in, 2 out]
                    n176 = Less?(x=w201, y=w202) -> (x < y?=w198:bool)
                    n177 = property on="Total 2D Histogram" class="IntGraph (strict)"() -> ("Value"=w197:dbl[][])  [unwired: 2 in, 2 out]
                    n178 = Index Array(array=w208, index=w205) -> (element=w204:bool)
                    n179 = property on="CurvesInHistogram" class="Arr (strict)"() -> ("Value"=w207:bool[])  [unwired: 2 in, 2 out]
                    n180 = Not(x=w204) -> (.not. x?=w203:bool)
                    n181 = case shown="True" w204 {
                      tunnel: w197 -> [w212 w215]
                      tunnel: w195 -> [w211 w214]
                      tunnel: [w210 w213] -> w196
                      frame #0 {
                        n182 = Add(x=w212, y=w211) -> (x+y=w210:dbl[][])
                      }
                      frame #1 {
                        n183 = Subtract(x=w215, y=w214) -> (x-y=w213:dbl[][])
                      }
                    }
                    n184 = Select(t=w201, s=w198, f=w200) -> (s? t:f=w199:i32)
                    n185 = Replace Array Subset(array=w207, new element=w203, index=w205) -> (w206:bool[])
                    n186 = property on="CurvesInHistogram" class="Arr (strict)"("Value"=w206) -> ()  [unwired: 2 in, 2 out]
                    n187 = property on="Add Histogram?" class="Bool (strict)"("Value"=FALSE ("Add Histogram?")) -> ()  [unwired: 2 in, 2 out]
                    n188 = property on="Total 2D Histogram" class="IntGraph (strict)"("Value"=w196) -> ()  [unwired: 2 in, 2 out]
                  }
                }
              }
              frame #1 {
                n189 = property on="Total 2D Histogram" class="IntGraph (strict)"() -> ("Value"=w217:dbl[][])  [unwired: 2 in, 2 out]
                n190 = property on="Individual 2D Histogram" class="IntGraph (strict)"() -> ("Value"=w218:dbl[][])  [unwired: 2 in, 2 out]
                n191 = property on="CurvesInHistogram" class="Arr (strict)"() -> ("Value"=w225:bool[])  [unwired: 2 in, 2 out]
                n192 = Increment(x=w224) -> (x+1=w220:i32)
                n193 = Less?(x=w220, y=w221) -> (x < y?=w219:bool)
                n194 = Add(x=w218, y=w217) -> (x+y=w216:dbl[][])
                n195 = Replace Array Subset(array=w225, new element=TRUE ("new element/subarray"), index=w224) -> (w222:bool[])
                n196 = property on="CurvesInHistogram" class="Arr (strict)"("Value"=w222) -> ()  [unwired: 2 in, 2 out]
                n197 = property on="1-D Histogram?" class="Bool (strict)"("Value"=TRUE ("1-D Histogram?")) -> ()  [unwired: 2 in, 2 out]
                n198 = property on="Total 2D Histogram" class="IntGraph (strict)"("Value"=w216) -> ()  [unwired: 2 in, 2 out]
                n199 = Select(t=w220, s=w219, f=w224) -> (s? t:f=w227:i32)
                n200 = property on="Continuous?" class="Bool (strict)"("Value"=w219) -> ()  [unwired: 2 in, 2 out]
              }
            }
          }
          frame #1 {
            # "Curve Browse:"
            n201 = case shown="False" w232 {
              tunnel: w231 -> [w234 w236]
              tunnel: [w233 w235] -> w230
              frame #0 {
                n202 = Increment(x=w234) -> (x+1=w233:i32)
              }
              frame #1 {
                n203 = Decrement(x=w236) -> (x-1=w235:i32)
              }
            }
            n204 = property on="Continuous?" class="Bool (strict)"("Value"=FALSE ("Continuous?")) -> ()  [unwired: 2 in, 2 out]
          }
        }
      }
    }
  }
